vi "Find Chessboard Corners.vi"   [LabVIEW 2020, in "g_ar_toolkit.camera_calibration.lvlib"]
uses:
  g_ar_toolkit.camera_calibration.lvlib
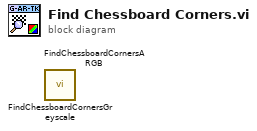
[diagram p0: block diagram]
diagram:
  n1 = call "FindChessboardCornersGreyscale.vi"() -> ()  [unwired: 9 in, 3 out]
  n2 = call "FindChessboardCornersARGB.vi"() -> ()  [unwired: 9 in, 3 out]
